vi "Throttle.vi"() -> ()   [LabVIEW 2011]
panel:
  in  "Mod1 2/AI9":fxp<+/-,26,5>
  out "Throttle Percent":fxp<+,14,1>
  in  "Throttle Max":fxp<+,16,4>
  in  "Throttle Min":fxp<+,16,4>
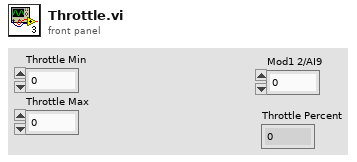
[diagram p1: front panel]
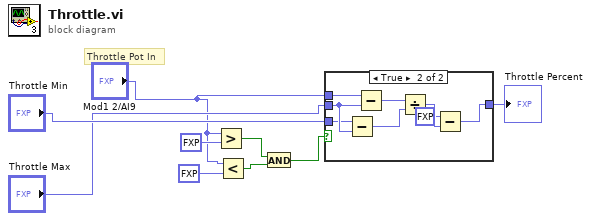
[diagram p0: block diagram]
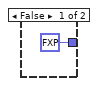
[diagram p2: hidden frame]
diagram:
  # "Throttle Pot In"
  n1 = Greater?(x="Mod1 2/AI9", y=fxp<+/-,26,5> 0.5) -> (0:w7:bool)
  n2 = Less?(x="Mod1 2/AI9", y=fxp<+/-,26,5> 5.5) -> (x < y?=w6:bool)
  n3 = And(x=w7, y=w6) -> (x .and. y?=w5:bool)
  n4 = case shown="True" w5 {
    tunnel: "Mod1 2/AI9" -> [_ w18]
    tunnel: "Throttle Max" -> [_ w16]
    tunnel: "Throttle Min" -> [_ w15]
    tunnel: [fxp<+/-,44,18> 0.0 w11] -> w9
    frame False {
    }
    frame True {
      n5 = Subtract(x=w15, y=w16) -> (x-y=w14:fxp<+/-,17,5>)
      n6 = Subtract(x=w18, y=w16) -> (x-y=w17:fxp<+/-,27,6>)
      n7 = Divide(x=w17, y=w14) -> (x/y=w13:fxp<+/-,44,18>)
      n8 = Subtract(x=fxp<+/-,44,18> 1.0, y=w13) -> (x-y=w11:fxp<+/-,45,19>)
    }
  }
  "Throttle Percent" <- w9
